vi "Configure Motor (Analog Speed).vi"(0 "VISA resource name":refnum<visa-resource-name>, 1 "Auto Range (F: Disable)":bool, 2 "Scaling Factor (1.0000)":dbl=1.0 min=0.0001 max=99999.9999 format="%.4f", 5 "Manual Range (20V)":i32(ring)=20 items=["1"=1, "2"=2, "5"=5, "10"=10, "20"=20], 7 "Linear Scale A (1.000)":dbl=1.0 min=0.001 max=1000000.0 format="%.3g", 9 "Linear Scale B (0.000)":dbl min=-1000000.0 max=1000000.0 format="%.3g", 11 "error in (no error)":errorcluster, 12 "Line Filter (0: OFF)":i32(ring) items=["OFF", "100", "1k"], 13 "Synchronization Source (13: None)":i32(ring)=13 items=["U1", "I1", "U2", "I2", "U3", "I3", "U4", "I4", "U5", "I5", "U6", "I6", "External Clock", "None"]) -> (4 "VISA resource name out":refnum<visa-resource-name>, 15 "error out":errorcluster)   [LabVIEW 2021, in "Yokogawa WT1800 Series.lvlib"]
doc: "Configures the analog speed motor features.\n\n<b>Note:</b>\nThis setting valid on models with the motor evaluation function (/MTR) option."
uses:
  <instrlib>/Yokogawa WT1800 Series/Yokogawa WT1800 Series.lvlib
panel:
  # "V"
  # "Hz"
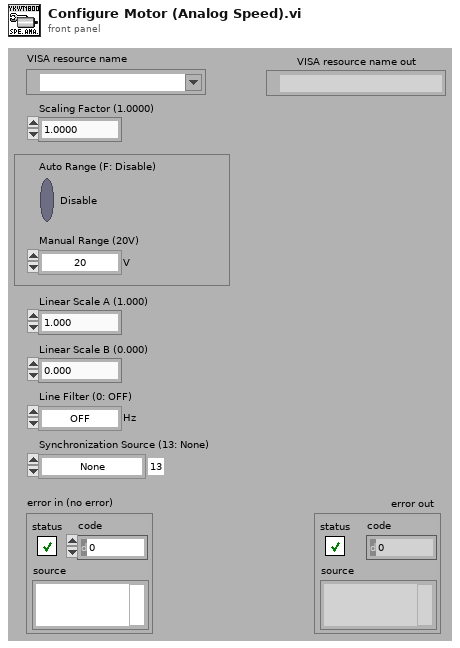
[diagram p1: front panel]
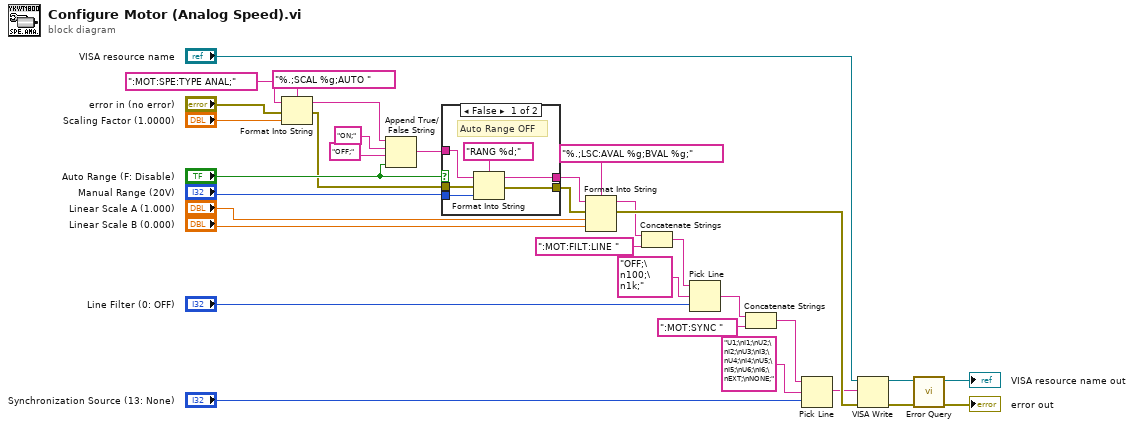
[diagram p0: block diagram]
diagram:
  n1 = Format Into String(format string="%.;SCAL %g;AUTO " ("形式文字列"), initial string=":MOT:SPE:TYPE ANAL;" ("形式文字列"), error in="error in (no error)", "Scaling Factor (1.0000)") -> (resulting string=w17:string, error out=w13:errorcluster)
  n2 = Append True/False String ("True/False 文字列を追加")(1:"Auto Range (F: Disable)", 2:"OFF;", 3:"ON;", 4:w17) -> (0:w16:string)
  n3 = case shown="False" "Auto Range (F: Disable)" {
    tunnel: w16 -> [w38 w40]
    tunnel: "Manual Range (20V)" -> [w37 _]
    tunnel: w13 -> [w36 w41]
    tunnel: [w35 w41] -> w11
    tunnel: [w34 w40] -> w10
    frame False {
      # "Auto Range OFF"
      n4 = Format Into String(format string="RANG %d;" ("形式文字列"), initial string=w38, error in=w36, w37) -> (resulting string=w34:string, error out=w35:errorcluster)
    }
    frame True {
      # "Auto Range ON"
    }
  }
  n5 = Format Into String(format string="%.;LSC:AVAL %g;BVAL %g;" ("形式文字列"), initial string=w10, error in=w11, "Linear Scale A (1.000)", "Linear Scale B (0.000)") -> (resulting string=w7:string, error out=w22:errorcluster)
  n6 = Concatenate Strings(w7, ":MOT:FILT:LINE " ("形式文字列")) -> (w6:string)
  n7 = Pick Line ("ライン選択")(string ("")=w6, multi-line string="OFF;\n100;\n1k;" ("複数行文字列"), line index="Line Filter (0: OFF)") -> (output string=w2:string)
  n8 = Concatenate Strings(w2, ":MOT:SYNC " ("形式文字列")) -> (w1:string)
  n9 = Pick Line ("ライン選択")(string ("")=w1, multi-line string="U1;\nI1;\nU2;\nI2;\nU3;\nI3;\nU4;\nI4;\nU5;\nI5;\nU6;\nI6;\nEXT;\nNONE;" ("複数行文字列"), line index="Synchronization Source (13: None)") -> (output string=w4:string)
  n10 = VISA Write ("VISA書き込み")(VISA resource name="VISA resource name", write buffer=w4, error in (no error)=w22) -> (VISA resource name out=w33:refnum<visa-resource-name>, error out=w32:errorcluster)  [unwired: 1 out]
  n11 = call <instrlib>:"Error Query.vi"("error in (no error)"=w32, "VISA resource name"=w33) -> ("error out"=→"error out":errorcluster, "VISA resource name out"=→"VISA resource name out":refnum<visa-resource-name>)  [unwired: 6 in, 2 out]
